vi "sig priority.vi"() -> ()   [LabVIEW 2020]
uses:
  <vilib>/Analysis/Matrix/Datatypes/RealMatrix.ctl
  <vilib>/Platform/TimedLoop/XDataNode/timing_clust.ctl
  <vilib>/Platform/TimedLoop/XDataNode/nitl_modes.ctl
  <vilib>/Platform/TimedLoop/XDataNode/wakeup.ctl
  <vilib>/Analysis/Matrix/Numeric/Conversions/Array To Matrix - RA.vi
  <vilib>/platform/TimedLoop/XDataNode/XDataNode.xnode
  <vilib>/Analysis/Matrix/NI_Matrix.lvlib
  <vilib>/Platform/TimedLoop/XDataNode/XDNodeRunTimeDep.lvlib
panel:
  out "overall time":u32
  out "product":T1
  in  "vector size":i32=20
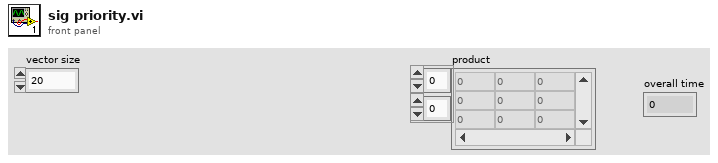
[diagram p1: front panel]
types:
  T1 = typedef "NI_Matrix.lvlib/RealMatrix.ctl" = dbl[][]
  T2 = typedef "XDNodeRunTimeDep.lvlib/timing_clust.ctl" = cluster{"Expected End [f-1]":u64, "Actual End [f-1]":u64, "Finished Late? [f-1]":bool, "Expected End [i-1]":u64, "Actual End [i-1]":u64, "Finished Late? [i-1]":bool, "Expected Start [i]":u64, "Actual Start [i]":u64, "Expected Start [f]":u64, "Actual Start [f]":u64, "Source Name":string, "Structure Name":string, "Period":i64, "Deadline":i64, "Offset":i64, "Start":i64, "Priority":i32, "Timeout":i32, "Mode":T3, "Wakeup Reason":T4, "Error":errorcluster, "Source Type":string, "Secondary Source Type":string, "Global End Time":u64, "Global Start Time":u64, "Frame Duration":u64, "Iteration Duration":u64, "Assigned CPU":i32, "I/O Scan Engine Mode":u32}
  T3 = typedef "XDNodeRunTimeDep.lvlib/nitl_modes.ctl" = enum32{"No Change", "Process missed periods, maintain original phase", "Discard missed periods, maintain original phase", "Process missed periods, ignore original phase", "Discard missed periods, ignore original phase"}
  T4 = typedef "XDNodeRunTimeDep.lvlib/wakeup.ctl" = enum32{"Normal", "Aborted", "Asynchronous wakeup", "Timing source error", "Timed loop error", "Timeout"}
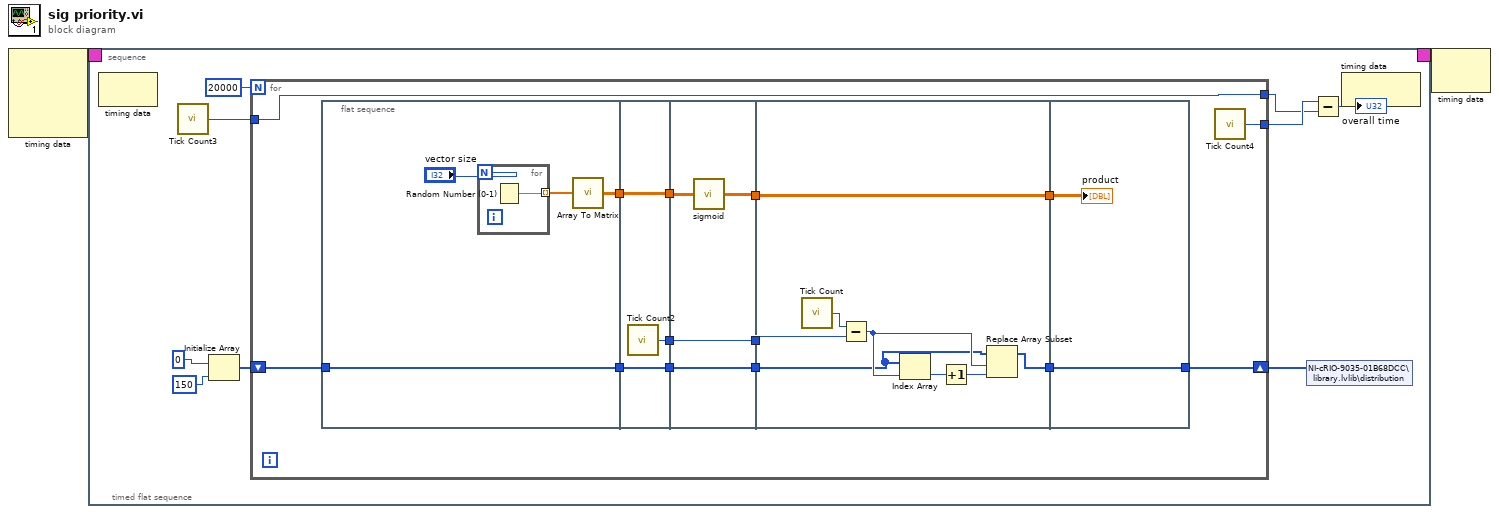
[diagram p0: block diagram]
diagram:
  n1 = node-c288() -> (w2:T2)  [unwired: 4 in]
  n2 = timed-sequence {
    timing: w2 -> [_]
    timing-out: [_] -> w1
    n3 = timed-flat-sequence {
      n4 = node-c288() -> ()  [unwired: 1 in, 1 out]
      n5 = call "Tick Count3"() -> ("Tick Count(uSec)"=w7:u32)
      n6 = Initialize Array(0, 150) -> (w8:i32[])
      n7 = for {
        N: 20000 -> [_]
        shift-right: [w14] -> w3
        shift-left: w8 -> [w16]
        tunnel: [w13] -> w5
        tunnel: w7 -> [w13]
        tunnel: [w12] -> w6
        n8 = flat-sequence {
          tunnel: [w28] -> w25
          tunnel: [w26] -> w17
          tunnel: w16 -> [w26]
          tunnel: w25 -> [w33]
          tunnel: [w33] -> w24
          tunnel: [w32] -> w23
          tunnel: [w31] -> w18
          tunnel: w17 -> [w31]
          tunnel: w24 -> [w34]
          tunnel: w23 -> [w37]
          tunnel: [w37] -> w22
          tunnel: [w35] -> w21
          tunnel: [w36] -> w19
          tunnel: w18 -> [w36]
          tunnel: w21 -> [w43]
          tunnel: w22 -> [w44]
          tunnel: [w43] -> w20
          tunnel: w19 -> [w39]
          tunnel: [w38] -> w15
          tunnel: w20 -> [w47]
          tunnel: w15 -> [w46]
          tunnel: [w46] -> w14
          frame #0 {
            n9 = for {
              N: "vector size" -> [_]
              tunnel: [w30] -> w29 mode=indexing
              n10 = Random Number (0-1)() -> (number: 0 to 1=w30:dbl)
            }
            n11 = call-poly <vilib>:"Array To Matrix.vi"("Real 1D Array"=w29) -> ("Real Matrix (Column Vector)"=w28:T1)
          }
          frame #1 {
            n12 = call "Tick Count2"() -> ("Tick Count(uSec)"=w32:u32)
          }
          frame #2 {
            n13 = call <vilib>:"sigmoid.vi"("x"=w34) -> ("y"=w35:T1)
          }
          frame #3 {
            n14 = call "Tick Count"() -> ("Tick Count(uSec)"=w45:u32)
            n15 = Subtract(x=w45, y=w44) -> (x-y=w40:u32)
            n16 = Index Array(array=w39, index=w40) -> (element=w41:i32)
            n17 = Increment(x=w41) -> (x+1=w42:i32)
            n18 = Replace Array Subset(array=w39, new element=w42, index=w40) -> (w38:i32[])
          }
          frame #4 {
            "product" <- w47
          }
        }
        n19 = call "Tick Count4"() -> ("Tick Count(uSec)"=w12:u32)
      }
      n20 = shared-variable "NI-cRIO-9035-01B68DCC\\library.lvlib\\distribution"(w3) -> ()  [unwired: 1 in, 1 out]
      n21 = Subtract(x=w6, y=w5) -> (x-y=→"overall time":u32)
      n22 = node-c288() -> ()  [unwired: 1 in, 1 out]
    }
  }
  n23 = node-c288(w1) -> ()  [unwired: 1 out]
